vi "Close.vi"(8 "error in (no error)":errorcluster, 11 "EventAPI in":refnum<class "EventAPI.lvclass">) -> (0 "error out":errorcluster, 3 "EventAPI out":refnum<class "EventAPI.lvclass">)   [LabVIEW 2020, in "Volatus.lvlib" / "EventAPI.lvclass"]
uses:
  EventAPI.lvclass
  EventAPI.lvclass/EventAPI.ctl
  <vilib>/ActorFramework/Stop Msg/Stop Msg.lvclass
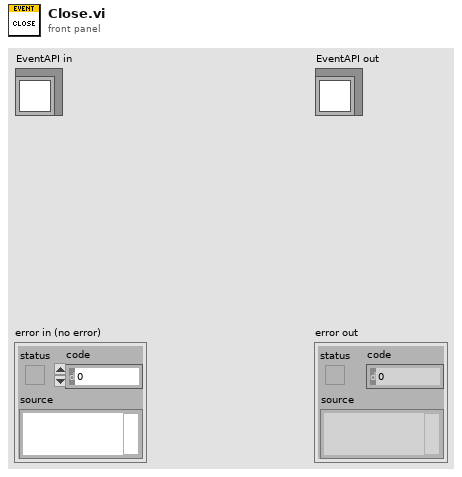
[diagram p1: front panel]
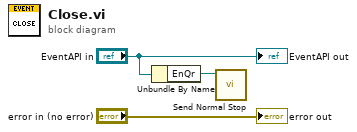
[diagram p0: block diagram]
diagram:
  n1 = Unbundle By Name("EventAPI in") -> ("EnQr"=w1:refnum<class "Message Enqueuer.lvclass">)
  n2 = call <vilib>:"Send Normal Stop.vi"("Message Enqueuer"=w1) -> ()  [unwired: 10 in, 1 out]
  "error out" <- "error in (no error)"
  "EventAPI out" <- "EventAPI in"
